vi "ControladorFCC.vi"() -> ()   [LabVIEW 2019]
uses:
  <vilib>/Analysis/Matrix/Datatypes/RealMatrix.ctl
  <vilib>/addons/control/pid/pid.llb/PID (DBL).vi
  <vilib>/addons/control/pid/NI_PID_pid.lvlib
  <vilib>/Analysis/Matrix/NI_Matrix.lvlib
panel:
  out "String Retardo":string
  in  "Retardo padé":dbl
  out "Error":dbl
  out "Lazo abierto":bool
  out "Lazo Cerrado":bool
  in  "Sp LC":dbl format="%.2f"
  in  "Estado":bool
  out "y(k)":dbl
  out "Salida del sistema":cluster{"y(k)":dbl, "ut":dbl}(graph)
  out "Den":string
  out "Num":string
  in  "Ut LA":dbl
  in  "dt":dbl
  in  "Denominador":dbl[](array[numeric])
  in  "Numerador":dbl[](array[numeric])
  # "Función de transferencia"
  # "x"
  # "sg"
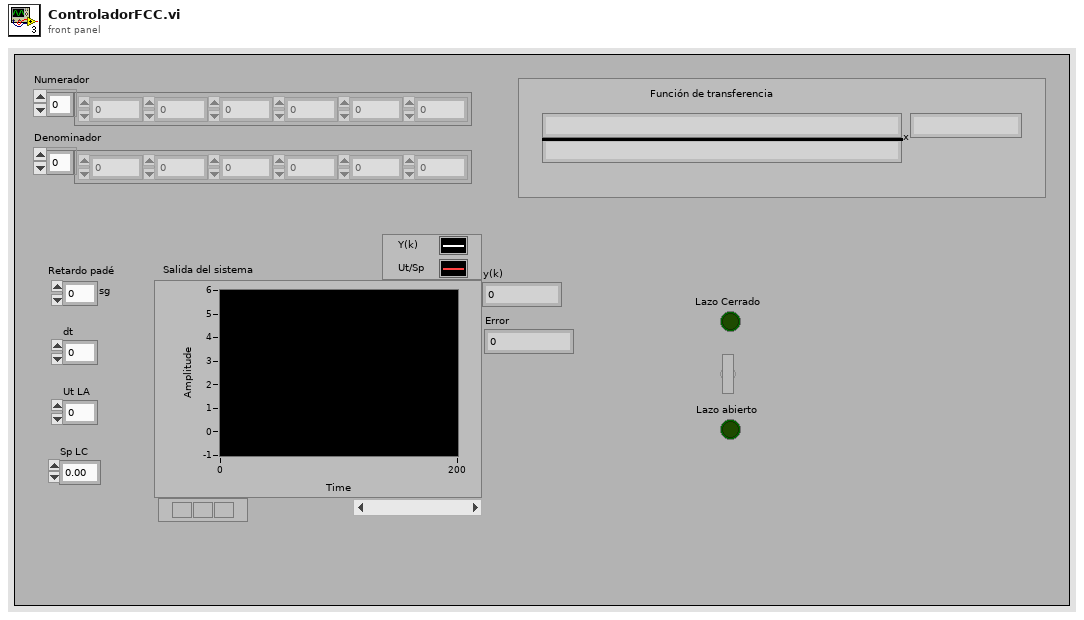
[diagram p1: front panel]
types:
  T1 = typedef "NI_Matrix.lvlib/RealMatrix.ctl" = dbl[][]
  T2 = cluster{"proportional gain (Kc)":dbl, "integral time (Ti, min)":dbl, "derivative time (Td, min)":dbl}
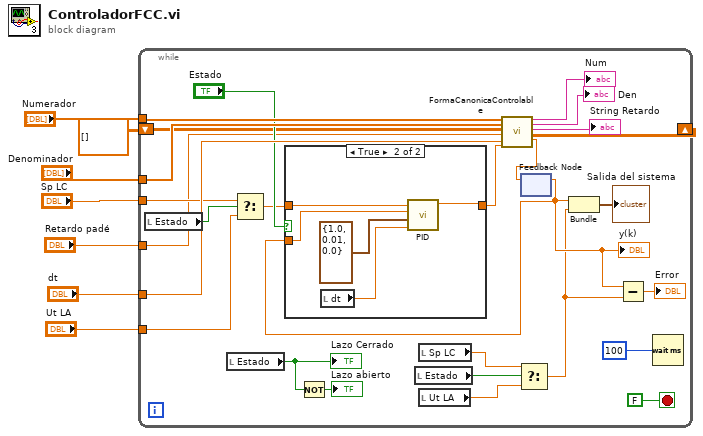
[diagram p0: block diagram]
diagram:
  n1 = while {
    tunnel: "Numerador" -> [w34]
    tunnel: "Denominador" -> [w26]
    shift-right: [w30] -> _
    shift-left: T1 [] ("x(k)") -> [w9]
    tunnel: "dt" -> [w33]
    tunnel: "Ut LA" -> [w22]
    tunnel: "Sp LC" -> [w23]
    tunnel: "Retardo padé" -> [w10]
    stop <- FALSE stop-if-true
    n2 = local read "Estado"() -> (w24:bool)
    n3 = local read "Estado"() -> (w18:bool)
    "Lazo Cerrado" <- w18
    n4 = Select(t=w23, s=w24, f=w22) -> (s? t:f=w21:dbl)
    n5 = Not(x=w18) -> (.not. x?=→"Lazo abierto":bool)
    n6 = local read "Estado"() -> (w14:bool)
    n7 = local read "Sp LC"() -> (w16:dbl)
    n8 = local read "Ut LA"() -> (w15:dbl)
    n9 = Select(t=w16, s=w14, f=w15) -> (s? t:f=w12:dbl)
    n10 = feedback #1() -> (w13:dbl)  [unwired: 1 in]
    "y(k)" <- w13
    n11 = case shown="True" "Estado" {
      tunnel: w21 -> [w35 w39]
      tunnel: [w35 w38] -> w20
      tunnel: w13 -> [_ w37]
      frame False {
      }
      frame True {
        n12 = local read "dt"() -> (w40:dbl)
        n13 = call-poly <vilib>:"PID.vi"("dt (s)"=w40, "PID gains"=T2 {"proportional gain (Kc)"=1.0, "integral time (Ti, min)"=0.01, "derivative time (Td, min)"=0.0}, "process variable"=w37, "setpoint"=w39) -> ("output"=w38:dbl)  [unwired: 6 in, 1 out]
      }
    }
    n14 = call "FormaCanonicaControlable.vi"("Num"=w34, "Den"=w26, "Xi"=w9, "Retardo padé"=w10, "dt"=w33, "u(k)"=w20) -> ("Num"=→"Num":string, "Den"=→"Den":string, "String Retardo"=→"String Retardo":string, "x(k)"=w30:T1, "y(k)"=w19:dbl)  [unwired: 9 in]
    n15 = feedback-in #1(w19) -> ()
    n16 = Bundle("y(k)"=w13, "Ut LA"=w12) -> (→"Salida del sistema":cluster{"y(k)":dbl, "Ut LA":dbl})  [unwired: 1 in]
    n17 = Subtract(x=w13, y=w12) -> (x-y=→"Error":dbl)
    n18 = Wait (ms)(milliseconds to wait=u32 100) -> ()  [unwired: 1 out]
  }
